vi "(SubVI)Update Voltage Range Ring Item.vi"(10 "error in (no error)":errorcluster caption="에러 입력(에러 없음)", 11 "Voltage Range Ring Ref (U8)":refnum<vi>) -> (2 "error out":errorcluster caption="에러 출력")   [LabVIEW 2020]
uses:
  Variables/(Var)System Variables.vi
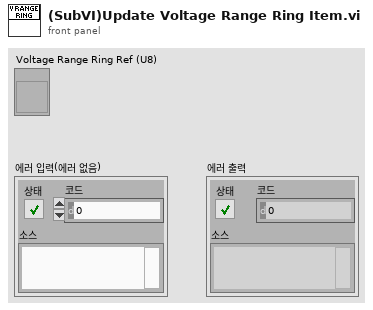
[diagram p1: front panel]
types:
  T1 = typedef "Haptic IC.lvclass/(Ctrl)IC Type.ctl" = enum8{"DW7800", "DW7912", "DW7914"}
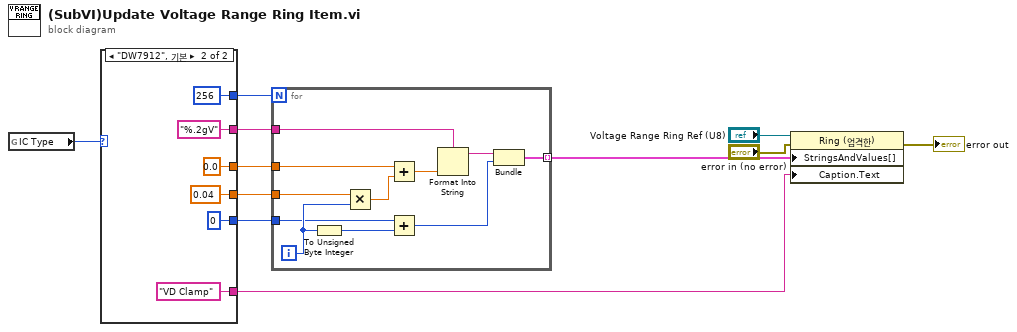
[diagram p0: block diagram]
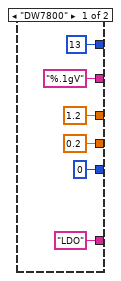
[diagram p2: hidden frame]
diagram:
  n1 = global read "(Var)System Variables.vi" "IC Type"() -> (w11:T1)
  n2 = case shown="\"DW7912\", 기본" w11 {
    tunnel: [13 256] -> w10
    tunnel: [1.2 0.0] -> w9
    tunnel: [0.2 0.04] -> w8
    tunnel: [u8 0 u8 0] -> w7
    tunnel: ["%.1gV" ("포맷 문자열") "%.2gV" ("포맷 문자열")] -> w2
    tunnel: ["LDO" "VD Clamp"] -> w1
    frame "DW7800" {
    }
    frame "DW7912", Default {
    }
  }
  n3 = for {
    N: w10 -> [_]
    tunnel: w9 -> [w32]
    tunnel: w8 -> [w34]
    tunnel: w7 -> [w29]
    tunnel: [w25] -> w6 mode=indexing
    tunnel: w2 -> [w24]
    i -> [w33]
    n4 = To Unsigned Byte Integer(number=w33) -> (unsigned 8bit integer=w30:u8)
    n5 = Multiply(x=w34, y=w33) -> (x*y=w31:dbl)
    n6 = Add(x=w32, y=w31) -> (x+y=w28:dbl)
    n7 = Add(x=w29, y=w30) -> (x+y=w26:u8)
    n8 = Format Into String(format string=w24, w28) -> (resulting string=w27:string)  [unwired: 2 in, 1 out]
    n9 = Bundle(w27, w26) -> (w25:cluster{string, u8})  [unwired: 1 in]
  }
  n10 = property class="Ring (엄격한)"(reference="Voltage Range Ring Ref (U8)", error in="error in (no error)", "StringsAndValues[]"=w6, "Caption.Text"=w1) -> (error out=→"error out":errorcluster)  [unwired: 1 out]
